vi "Authorization.vi"() -> (3 "SetAuthorizationCode":bool)   [LabVIEW 2020, in "HslCommunication.lvlib"]
uses:
  HslCommunication.lvlib
  E:/Git/Libraries/develop/HslCommunication/_Dependenciecs/HslCommunication.dll
  _Dependenciecs/HslCommunication.dll
panel:
  out "error out":errorcluster
  in  "error in (no error)":errorcluster
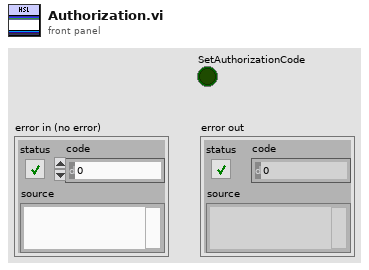
[diagram p1: front panel]
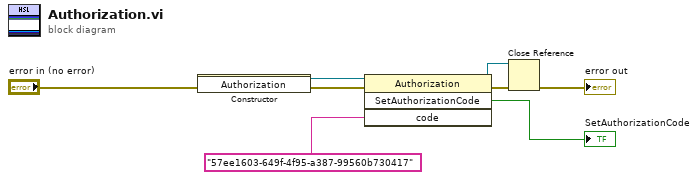
[diagram p0: block diagram]
diagram:
  n1 = constructor class="Authorization" ("Constructor Node")(error in="error in (no error)") -> (reference out=w1:refnum<k24>, error out=w5:errorcluster)  [unwired: 2 in, 1 out]
  n2 = invoke class="Authorization" method="SetAuthorizationCode"(reference=w1, error in=w5, "code"="57ee1603-649f-4f95-a387-99560b730417") -> (reference out=w7:refnum<k24>, error out=w8:errorcluster, "SetAuthorizationCode"=→"SetAuthorizationCode":bool)  [unwired: 1 in, 1 out]
  n3 = Close Reference(reference=w7, error in (no error)=w8) -> (error out=→"error out":errorcluster)
